vi "Set Current Limit.vi"(8 "error in (no error)":errorcluster, 10 "Current Limit (A)":dbl, 11 "Keysight_PSU in":refnum<class "Keithley_PSU.lvclass">) -> (0 "error out":errorcluster, 3 "Keysight_PSU out":refnum<class "Keithley_PSU.lvclass">)   [LabVIEW 2024, in "HAL_Example.lvlib" / "Keithley_PSU.lvclass"]
uses:
  Keithley_PSU.lvclass
  PSU/PSU.lvclass
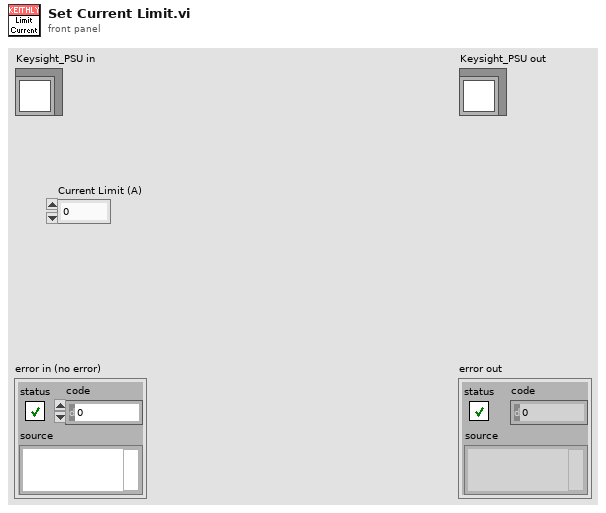
[diagram p1: front panel]
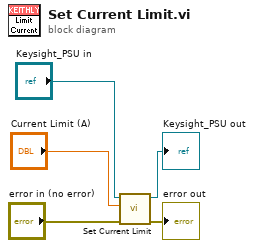
[diagram p0: block diagram]
diagram:
  n1 = call-parent "Set Current Limit.vi"("error in (no error)"="error in (no error)", "Current Limit (A)"="Current Limit (A)", "PSU in"="Keysight_PSU in") -> ("error out"=→"error out":errorcluster, "PSU out"=→"Keysight_PSU out":refnum<class "Keithley_PSU.lvclass">)  [unwired: 7 in]
